vi "ViHandler.RegisterVi.Main.vi"(8 "ErrorIn":errorcluster, 11 "ViInfo":T1) -> (0 "ErrorOut":errorcluster)   [LabVIEW 2016, in "ViHandler.lvclass"]
uses:
  ViHandler.lvclass
  ViHandler.ViInfo.ctl
  ObjectHandler/ObjectHandler.GetObjectWType.ctl
  ObjectHandler/ObjectHandler.ObjectWType.ctl
  ObjectHandler/ObjectHandler.ObjectType.ctl
  ObjectHandler/ObjectHandler.lvclass
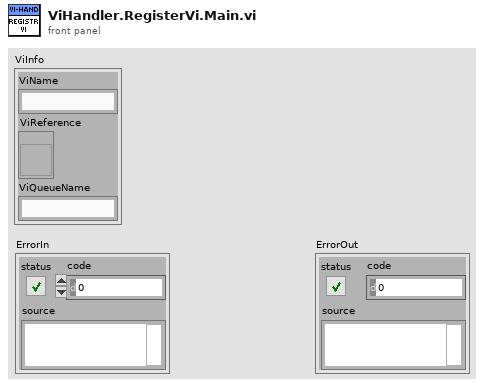
[diagram p1: front panel]
types:
  T1 = typedef "ViHandler.lvclass/ViHandler.ViInfo.ctl" = cluster{"ViName":string, "ViReference":refnum<vi>, "ViQueueName":string}
  T2 = typedef "ObjectHandler.lvclass/ObjectHandler.GetObjectWType.ctl" = cluster{"Name":string, "Caller":string}
  T3 = typedef "ObjectHandler.lvclass/ObjectHandler.ObjectWType.ctl" = cluster{"ObjectType":T4, "Object":variant}
  T4 = typedef "ObjectHandler.lvclass/ObjectHandler.ObjectType.ctl" = enum16{"undefined", "ObjectHandler", "ViHandler", "ErrorHandler", "CentralStorage", "Hausmodell", "Sondenmodell", "Wärmepumpe", "Umgebung"}
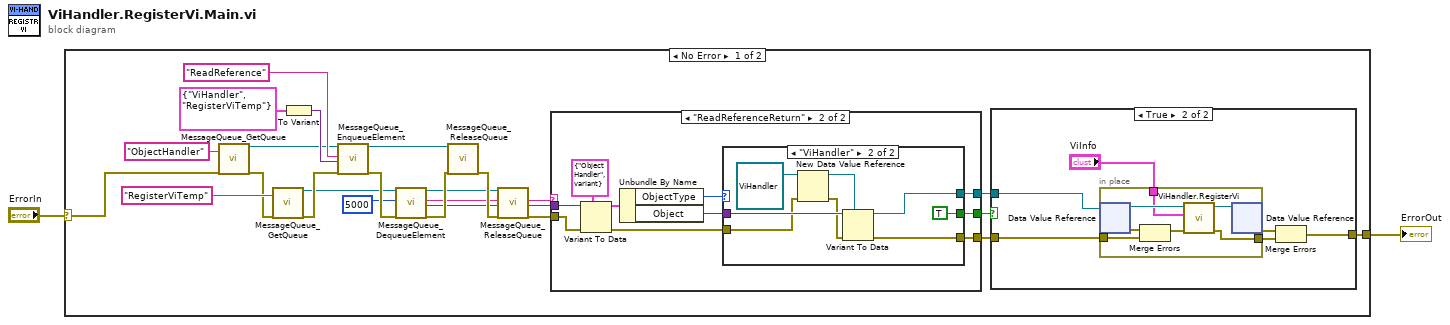
[diagram p0: block diagram]
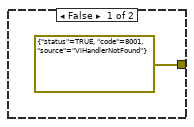
[diagram p2: hidden frame]
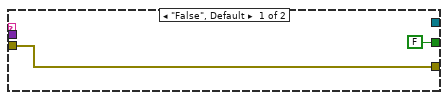
[diagram p3: hidden frame]
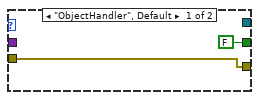
[diagram p4: hidden frame]
diagram:
  n1 = case shown="No Error" "ErrorIn" {
    selector: "ErrorIn" -> [w4 w62]
    tunnel: [w5 w62] -> w2
    frame No Error {
      n2 = call "MessageQueue_GetQueue.vi"("Name"="ObjectHandler", "ErrorIn"=w4) -> ("QueueOut"=w9:refnum<queue>, "ErrorOut"=w10:errorcluster)  [unwired: 15 in, 1 out]
      n3 = call "MessageQueue_GetQueue.vi"("Name"="RegisterViTemp" ("Caller"), "ErrorIn"=w10) -> ("QueueOut"=w15:refnum<queue>, "ErrorOut"=w19:errorcluster)  [unwired: 15 in, 1 out]
      n4 = To Variant(anything=T2 {"Name"="ViHandler", "Caller"="RegisterViTemp"} ("GetRefInput")) -> (Variant=w20:variant)
      n5 = call "MessageQueue_EnqueueElement.vi"("QueueIn"=w9, "Message"="ReadReference", "Data"=w20, "ErrorIn"=w19) -> ("QueueOut"=w12:refnum<queue>, "ErrorOut"=w17:errorcluster)  [unwired: 14 in]
      n6 = call "MessageQueue_DequeueElement.vi"("QueueIn"=w15, "Timeout"=5000, "ErrorIn"=w17) -> ("QueueOut"=w11:refnum<queue>, "Message"=w14:string, "Data"=w13:variant, "ErrorOut"=w25:errorcluster)  [unwired: 12 in, 1 out]
      n7 = call "MessageQueue_ReleaseQueue.vi"("QueueIn"=w12, "ErrorIn"=w25) -> ("ErrorOut"=w24:errorcluster)  [unwired: 15 in, 2 out]
      n8 = call "MessageQueue_ReleaseQueue.vi"("QueueIn"=w11, "ErrorIn"=w24) -> ("ErrorOut"=w8:errorcluster)  [unwired: 15 in, 2 out]
      n9 = case shown="\"ReadReferenceReturn\"" w14 {
        tunnel: w13 -> [_ w51]
        tunnel: [w40 w47] -> w7
        tunnel: w8 -> [w40 w45]
        tunnel: [FALSE w43] -> w6
        tunnel: [_ w42] -> w3
        frame "False", Default {
        }
        frame "ReadReferenceReturn" {
          n10 = Variant To Data(error in=w45, type=T3 {"ObjectType"=enum."ObjectHandler", "Object"=variant} ("ObjectWType"), Variant=w51) -> (data=w50:T3, error out=w44:errorcluster)
          n11 = Unbundle By Name(w50) -> ("ObjectType"=w49:T4, "Object"=w48:variant)
          n12 = case shown="\"ViHandler\"" w49 {
            tunnel: w48 -> [_ w61]
            tunnel: [w52 w58] -> w47
            tunnel: w44 -> [w52 w57]
            tunnel: [FALSE TRUE] -> w43
            tunnel: [_ w54] -> w42
            frame "ObjectHandler", Default {
            }
            frame "ViHandler" {
              n13 = New Data Value Reference(data value=refnum<class "ViHandler.lvclass"> refnum ("ViHandler.lvclass"), error in=w57) -> (data value reference=w59:refnum<data-value>, error out=w56:errorcluster)
              n14 = Variant To Data(error in=w56, type=w59, Variant=w61) -> (data=w54:refnum<data-value>, error out=w58:errorcluster)
            }
          }
        }
      }
      n15 = case shown="True" w6 {
        tunnel: w7 -> [_ w30]
        tunnel: [errorcluster {"status"=TRUE, "code"=8001, "source"="ViHandlerNotFound"} ("error IO") w29] -> w5
        tunnel: w3 -> [_ w27]
        frame False {
        }
        frame True {
          n16 = in-place {
            in-place-border: [w36] -> w32
            in-place-border: w30 -> [w34]
            in-place-border: "ViInfo" -> [w33]
            n17 = in-place-dvr #1(w27) -> (w38:refnum<class "ViHandler.lvclass">, w37:errorcluster)
            n18 = Merge Errors(w37, w34) -> (w35:errorcluster)
            n19 = call "ViHandler.RegisterVi.vi"("error in (no error)"=w35, "ViInfo"=w33, "ViHandler in"=w38) -> ("error out"=w36:errorcluster, "ViHandler out"=w39:refnum<class "ViHandler.lvclass">)  [unwired: 7 in]
            n20 = in-place-dvr #1(w39) -> (w31:errorcluster)  [unwired: 1 out]
          }
          n21 = Merge Errors(w31, w32) -> (w29:errorcluster)
        }
      }
    }
    frame Error {
    }
  }
  "ErrorOut" <- w2
